vi "is_a_letter.vi"(10 "String":string) -> (2 "is a letter":bool)   [LabVIEW 2013]
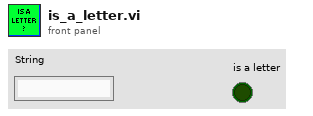
[diagram p1: front panel]
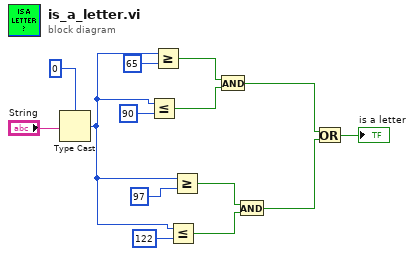
[diagram p0: block diagram]
diagram:
  n1 = Type Cast(type=u8 0, x="String") -> (*(type *) &x=w4:u8)
  n2 = Less Or Equal?(x=w4, y=u8 90) -> (x <= y?=w9:bool)
  n3 = Greater Or Equal?(x=w4, y=u8 65) -> (x >= y?=w10:bool)
  n4 = Less Or Equal?(x=w4, y=u8 122) -> (x <= y?=w8:bool)
  n5 = Greater Or Equal?(x=w4, y=u8 97) -> (x >= y?=w7:bool)
  n6 = And(x=w10, y=w9) -> (x .and. y?=w3:bool)
  n7 = And(x=w7, y=w8) -> (x .and. y?=w2:bool)
  n8 = Or(x=w3, y=w2) -> (x .or. y?=→"is a letter":bool)
